vi "Emballage_BDD_Enlever_doublon_Tableau.vi"(1 "Tableau_IN":string[](array[string])) -> (0 "Tableau_OUT":string[](array[string]))   [LabVIEW 2020]
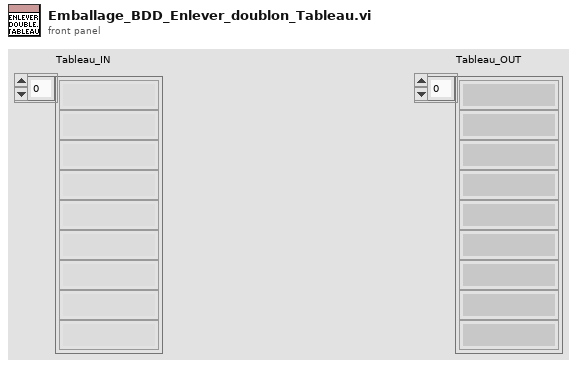
[diagram p1: front panel]
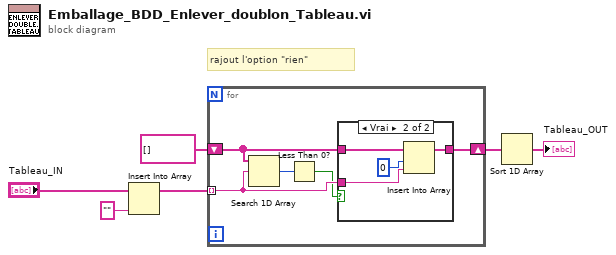
[diagram p0: block diagram]
diagram:
  # "rajout l'option \"rien\""
  n1 = Insert Into Array(array="Tableau_IN", new element="" ("nouvel élément/sous-tableau")) -> (w3:string[])  [unwired: 1 in]
  n2 = for {
    tunnel: w3 -> [w9] mode=indexing
    shift-right: [w11] -> w6
    shift-left: string[] [] -> [w10]
    n3 = Search 1D Array(1D array=w10, element=w9) -> (index of element=w8:i32)  [unwired: 1 in]
    n4 = Less Than 0?(x=w8) -> (x < 0?=w7:bool)
    n5 = case shown="Vrai" w7 {
      tunnel: [w12 w16] -> w11
      tunnel: w10 -> [w12 w15]
      tunnel: w9 -> [_ w14]
      frame False {
      }
      frame True {
        n6 = Insert Into Array(array=w15, index=0 ("indice"), new element=w14) -> (w16:string[])
      }
    }
  }
  n7 = Sort 1D Array(array=w6) -> (sorted array=→"Tableau_OUT":string[])
